vi "TCP-serial.vi"() -> ()   [LabVIEW 2016]
panel:
  out "Iteration":i32
  in  "Loop multiple (ms)":u32=500
  in  "remote port":u16=967
  in  "address":string="192.168.1.160"
  in  "stop":bool
  out "field value":string
  out "error out":errorcluster
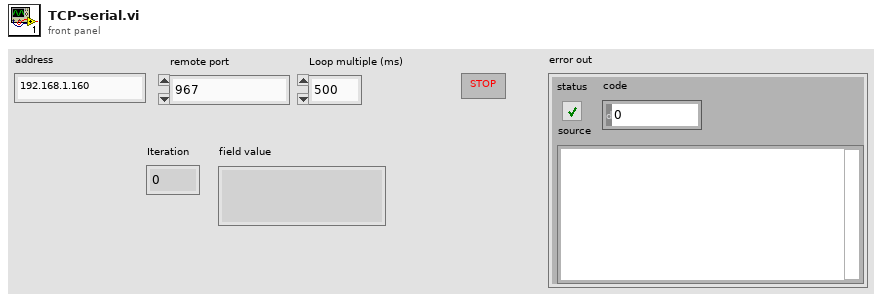
[diagram p1: front panel]
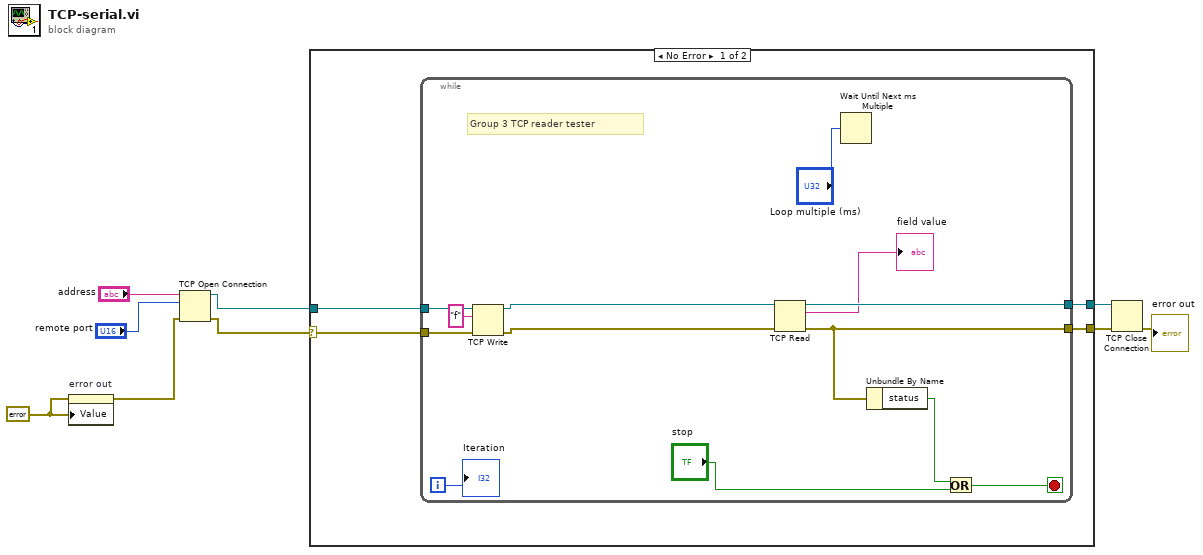
[diagram p0: block diagram]
diagram:
  w2 = errorcluster {"status"=FALSE, "code"=0, "source"=""} ("error in (no error)")
  n1 = property on="error out" class="Clust (strict)"(error in=w2, "Value"=w2) -> (error out=w3:errorcluster)  [unwired: 1 in, 1 out]
  n2 = TCP Open Connection(address="address", remote port or service name="remote port", error in (no error)=w3) -> (connection ID=w9:refnum<k5>, error out=w1:errorcluster)  [unwired: 2 in]
  n3 = case shown="No Error" w1 {
    selector: w1 -> [w10 _]
    tunnel: w9 -> [w13 w27]
    tunnel: [w12 w27] -> w8
    tunnel: [w11 _] -> w7
    frame No Error {
      n4 = while {
        tunnel: w13 -> [w25]
        tunnel: [w23] -> w12
        tunnel: w10 -> [w22]
        tunnel: [w18] -> w11
        i -> [w14]
        stop <- w16 stop-if-true
        # "Group 3 TCP reader tester"
        n5 = TCP Write(connection ID=w25, data in="f", error in (no error)=w22) -> (connection ID out=w24:refnum<k5>, error out=w21:errorcluster)  [unwired: 1 in, 1 out]
        n6 = TCP Read(connection ID=w24, error in (no error)=w21) -> (connection ID out=w23:refnum<k5>, data out=→"field value":string, error out=w18:errorcluster)  [unwired: 3 in]
        n7 = Wait Until Next ms Multiple(millisecond multiple="Loop multiple (ms)") -> ()  [unwired: 1 out]
        n8 = Unbundle By Name(w18) -> ("status"=w17:bool)
        n9 = Or(x=w17, y="stop") -> (x .or. y?=w16:bool)
        "Iteration" <- w14
      }
    }
    frame Error {
    }
  }
  n10 = TCP Close Connection(connection ID=w8, error in (no error)=w7) -> (error out=→"error out":errorcluster)  [unwired: 1 in, 1 out]
